vi "Read Current Status from Status Bar.vi"(9 "Status Bar":refnum<vi>) -> (0 "Current Status String":string, 1 "Status Bar Out":refnum<vi>)   [LabVIEW 2011]
panel:
  out "error out":errorcluster
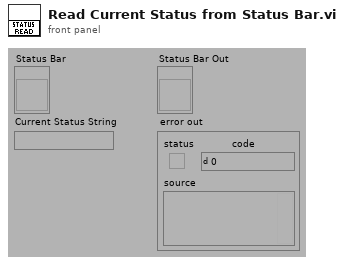
[diagram p1: front panel]
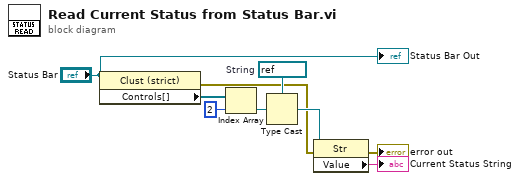
[diagram p0: block diagram]
diagram:
  w5 = refnum<vi> refnum  # String
  n1 = property class="Clust (strict)"(reference="Status Bar") -> (error out=w1:errorcluster, "Controls[]"=w3:refnum<vi>[])  [unwired: 1 in, 1 out]
  n2 = Index Array(array=w3, index=2) -> (element=w4:refnum<vi>)
  n3 = Type Cast(type=w5, x=w4) -> (*(type *) &x=w2:refnum<vi>)
  n4 = property class="Str"(reference=w2, error in=w1) -> (error out=→"error out":errorcluster, "Value"=→"Current Status String":string)  [unwired: 1 out]
  "Status Bar Out" <- "Status Bar"
